vi "IECMemory.UseOldMM.vi"(0 "i ref in":refnum<vi>, 3 "ms timeout (100)":i32=100, 5 "error in (no error)":errorcluster) -> (14 "i ref out":refnum<vi>, 16 "Use Old MM?":bool, 17 "timed out":bool, 19 "error out":errorcluster)   [LabVIEW 2014, in "IECMemory.lvlib"]
doc: "Gets the information from the data base if you want to use the old MM (new means MM6)."
uses:
  IECMemory.lvlib
  CSCore/BaseProcess/BaseProcess.lvlib
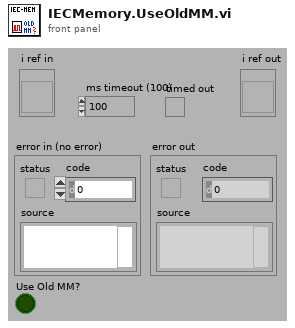
[diagram p1: front panel]
types:
  T1 = typedef "BaseProcess.lvlib/BaseProcess.i attribute.ctl" = cluster{"EventStatus":string, "EventError":i32, "PresetEvtWatchD":i32, "PresetPdcWatchD":i32, "EventTimeout":i32, "PeriodicInterval":i32, "Interface":string[], "Address":string[], "Special":string[], "PeriodicError":i32, "PeriodicStatus":string, "SuperProc":string, "Descriptors":T2[], "CaseRef":refnum<vi>, "PdcRef":refnum<vi>, "Thread Ref":refnum<vi>, "eventErrorID":i32, "eventStatusID":i32, "periodicErrorID":i32, "periodicStatusID":i32, "pdcCtrID":i32}
  T2 = typedef "BaseProcess.lvlib/BaseProcess.descriptor definition.ctl" = cluster{"selector":string, "descriptor":T3}
  T3 = typedef "BaseProcess.lvlib/BaseProcess.descriptor string definition.ctl" = string
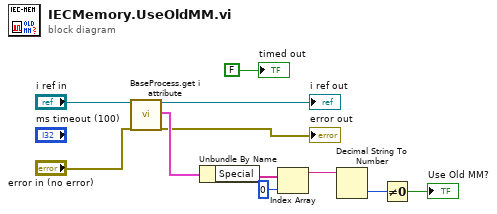
[diagram p0: block diagram]
diagram:
  n1 = call "BaseProcess.get i attribute.vi"("i ref in"="i ref in", "error in (no error)"="error in (no error)") -> ("i ref out"=→"i ref out":refnum<vi>, "i attribute"=w9:T1, "error out"=→"error out":errorcluster)  [unwired: 15 in]
  n2 = Unbundle By Name(w9) -> ("Special"=w8:string[])
  n3 = Index Array(array=w8, index=0 ("Index")) -> (element=w6:string)
  n4 = Decimal String To Number(string=w6) -> (number=w2:i32)  [unwired: 2 in, 1 out]
  n5 = Not Equal To 0?(x=w2) -> (x != 0?=→"Use Old MM?":bool)
  "timed out" <- FALSE ("timed out")
